vi "testSTRING Passes If Element Is Found.vi"(8 "error in (no error)":errorcluster, 11 "TestCase in":refnum<class "Search In 1D Array Test Case.lvclass">) -> (0 "error out":errorcluster, 3 "TestCase out":refnum<class "Search In 1D Array Test Case.lvclass">)   [LabVIEW 2015, in "Search In 1D Array Test Case.lvclass"]
uses:
  Search In 1D Array Test Case.lvclass
  SubVIs/Search in array/Pass If In 1D Array (STRING).vi
  <vilib>/addons/_JKI Toolkits/VI Tester/TestCase.llb/TestCase.lvclass
  VITAC.lvlib
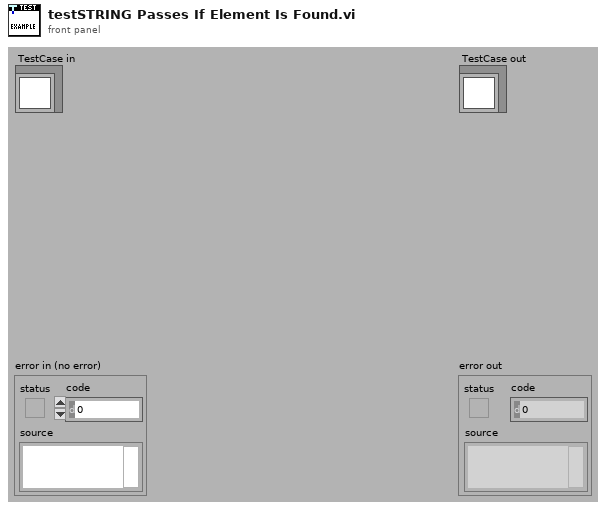
[diagram p1: front panel]
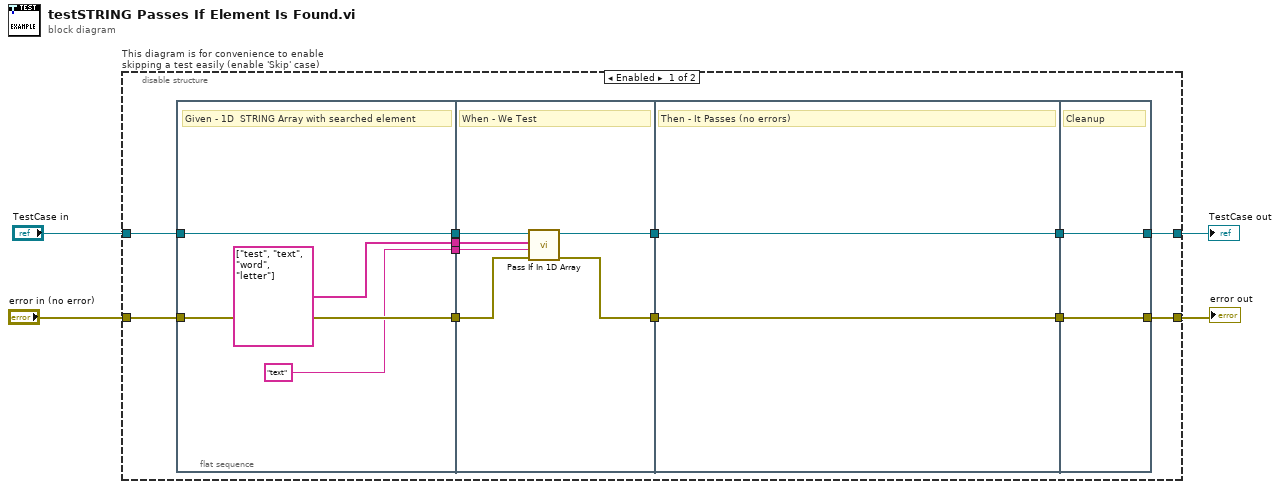
[diagram p0: block diagram]
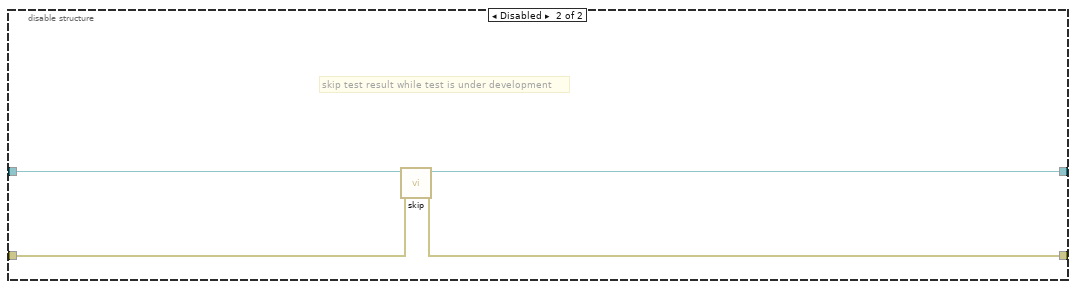
[diagram p2: hidden frame]
diagram:
  n1 = disable-structure "This diagram is for convenience to enable skipping a test easily (enable 'Skip' case)" shown="Enabled" {
    disable-tunnel: "TestCase in" -> [w8 w34]
    disable-tunnel: [w11 w32] -> w1
    disable-tunnel: [w10 w33] -> w3
    disable-tunnel: "error in (no error)" -> [w9 w31]
    frame Enabled {
      n2 = flat-sequence {
        tunnel: w9 -> [w19]
        tunnel: w8 -> [w20]
        tunnel: [w20] -> w16
        tunnel: [w19] -> w15
        tunnel: ["text"] -> w6
        tunnel: [string[] ["test", "text", "word", "letter"]] -> w5
        tunnel: [w25] -> w14
        tunnel: [w24] -> w13
        tunnel: w16 -> [w26]
        tunnel: w15 -> [w23]
        tunnel: w6 -> [w22]
        tunnel: w5 -> [w21]
        tunnel: [w28] -> w12
        tunnel: w14 -> [w28]
        tunnel: w13 -> [w27]
        tunnel: [w27] -> w7
        tunnel: [w29] -> w10
        tunnel: [w30] -> w11
        tunnel: w12 -> [w30]
        tunnel: w7 -> [w29]
        frame #0 {
          # "Given - 1D  STRING Array with searched element"
        }
        frame #1 {
          # "When - We Test"
          n3 = call-poly "Pass If In 1D Array.vi"("error in (no error)"=w23, "element"=w22, "1D array"=w21, "TestCase in"=w26) -> ("error out"=w24:errorcluster, "TestCase out"=w25:refnum<class "Search In 1D Array Test Case.lvclass">)  [unwired: 6 in]
        }
        frame #2 {
          # "Then - It Passes (no errors)"
        }
        frame #3 {
          # "Cleanup"
        }
      }
    }
    frame Disabled {
      # "skip test result while test is under development"
      n4 = call <vilib>:"skip.vi"("error in (no error)"=w31, "TestCase in"=w34) -> ("error out"=w33:errorcluster, "TestCase out"=w32:refnum<class "Search In 1D Array Test Case.lvclass">)  [unwired: 8 in]
    }
  }
  "error out" <- w3
  "TestCase out" <- w1
